vi "Enqueue Message.vi"(6 "우선순위 메시지?":bool, 8 "에러 입력(에러 없음)":errorcluster, 9 "값":variant, 10 "메세지":string, 11 "큐 입력":refnum<queue>) -> (0 "에러 출력":errorcluster, 3 "큐 출력":refnum<queue>)   [LabVIEW 2020]
uses:
  Controls/Message Cluster.ctl
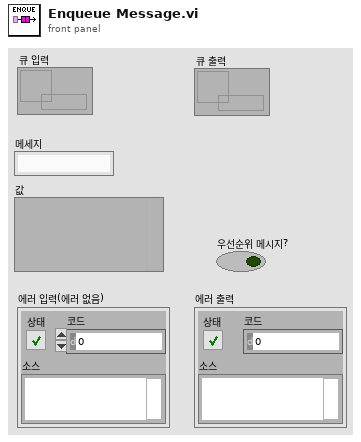
[diagram p1: front panel]
types:
  T1 = typedef "Message Cluster.ctl" = cluster{"메세지":string, "값":variant}
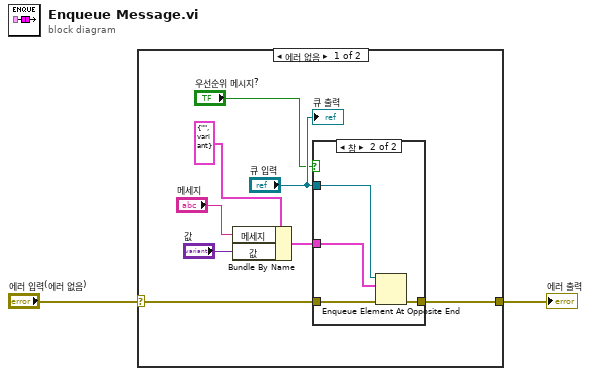
[diagram p0: block diagram]
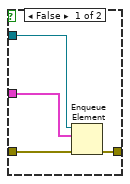
[diagram p2: hidden frame]
diagram:
  n1 = case shown="에러 없음" "에러 입력(에러 없음)" {
    selector: "에러 입력(에러 없음)" -> [w3 w19]
    tunnel: [w9 w19] -> w2
    frame No Error {
      n2 = Bundle By Name(cluster=T1 {"메세지"="", "값"=variant} ("원소"), "메세지"="메세지", "값"="값") -> (w7:T1)
      n3 = case shown="참" "우선순위 메시지?" {
        tunnel: "큐 입력" -> [w14 w18]
        tunnel: [w13 w17] -> w9
        tunnel: w3 -> [w12 w16]
        tunnel: w7 -> [w11 w15]
        frame False {
          n4 = Enqueue Element(queue=w14, element=w11, error in (no error)=w12) -> (error out=w13:errorcluster)  [unwired: 1 in, 2 out]
        }
        frame True {
          n5 = Enqueue Element At Opposite End(queue=w18, element=w15, error in (no error)=w16) -> (error out=w17:errorcluster)  [unwired: 1 in, 2 out]
        }
      }
      "큐 출력" <- "큐 입력"
    }
    frame Error {
    }
  }
  "에러 출력" <- w2
